vi "LHF.DB.Mongo.Bson.Waveform.vi"(0 "waveform":waveform(dbl), 5 "error in (no error)":errorcluster) -> (14 "BsonDocument":refnum<k24>, 19 "error out":errorcluster)   [LabVIEW 2013, in "LHF.DB.Mongo.lvclass"]
uses:
  LHF.DB.Mongo.lvclass
  C:/Users/Ricardo/Desktop/Projetos/LabVIEW-MongoDB/src/Driver/MongoDB.Bson.dll
  Driver/MongoDB.Bson.dll
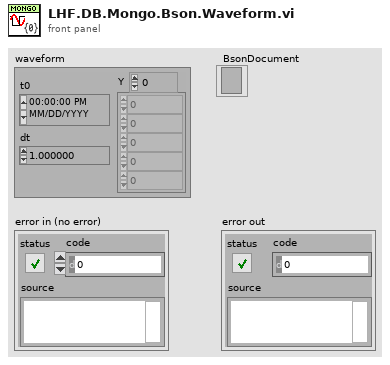
[diagram p1: front panel]
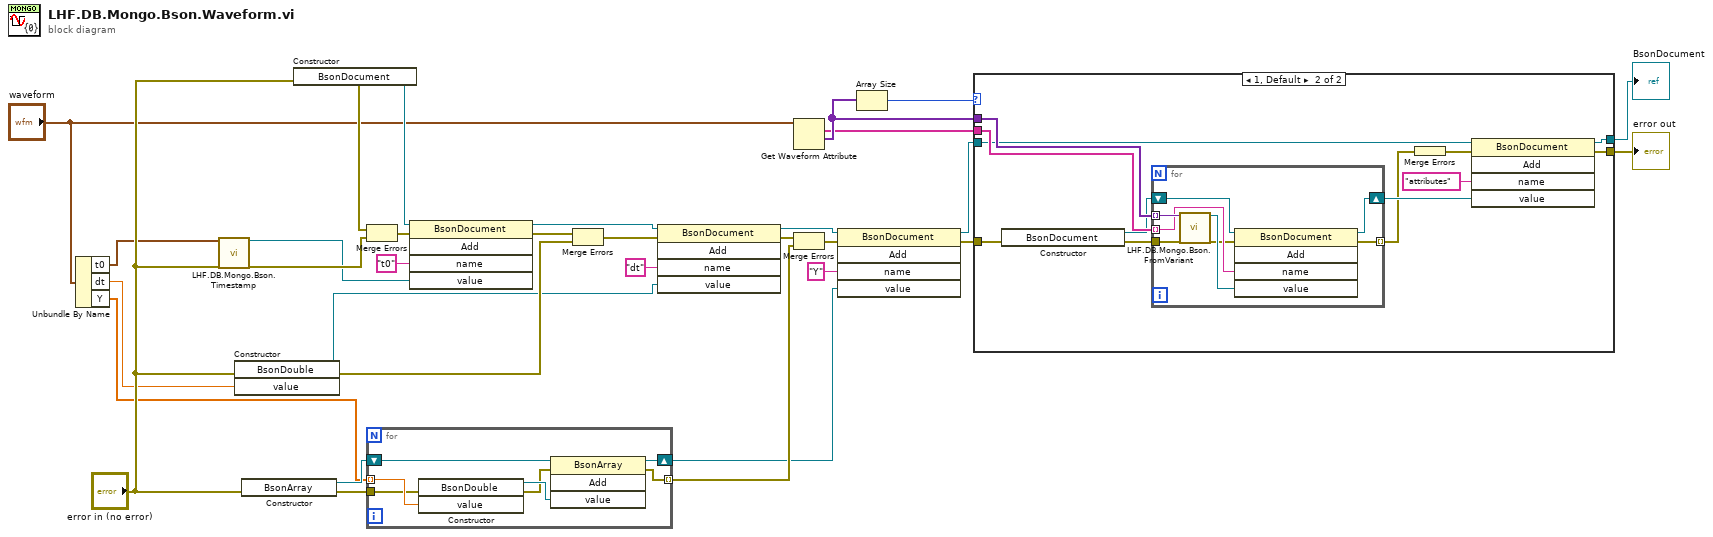
[diagram p0: block diagram]
diagram:
  n1 = Unbundle By Name("waveform") -> ("t0"=w5:timestamp, "dt"=w9:dbl, "Y"=w16:dbl[])
  n2 = call "LHF.DB.Mongo.Bson.Timestamp.vi"("t0"=w5, "error in (no error)"="error in (no error)") -> ("BsonString"=w8:refnum<k24>, "error out"=w25:errorcluster)  [unwired: 16 in]
  n3 = constructor class="BsonDouble"(error in="error in (no error)", "value"=w9) -> (reference out=w12:refnum<k24>, error out=w24:errorcluster)  [unwired: 2 in, 2 out]
  n4 = constructor class="BsonArray"(error in="error in (no error)") -> (reference out=w17:refnum<k24>, error out=w26:errorcluster)  [unwired: 2 in, 1 out]
  n5 = constructor class="BsonDocument"(error in="error in (no error)") -> (reference out=w6:refnum<k24>, error out=w31:errorcluster)  [unwired: 2 in, 1 out]
  n6 = Merge Errors(w31, w25) -> (w30:errorcluster)
  n7 = for {
    tunnel: w16 -> [w39] mode=indexing
    shift-right: [w36] -> w18
    shift-left: w17 -> [w38]
    tunnel: [w35] -> w22 mode=indexing
    tunnel: w26 -> [w34]
    n8 = constructor class="BsonDouble"(error in=w34, "value"=w39) -> (reference out=w37:refnum<k24>, error out=w33:errorcluster)  [unwired: 2 in, 2 out]
    n9 = invoke class="BsonArray" method="Add"(reference=w38, error in=w33, "value"=w37) -> (reference out=w36:refnum<k24>, error out=w35:errorcluster)  [unwired: 1 in, 2 out]
  }
  n10 = invoke class="BsonDocument" method="Add"(reference=w6, error in=w30, "name"="t0", "value"=w8) -> (reference out=w11:refnum<k24>, error out=w28:errorcluster)  [unwired: 1 in, 3 out]
  n11 = Merge Errors(w28, w24) -> (w27:errorcluster)
  n12 = invoke class="BsonDocument" method="Add"(reference=w11, error in=w27, "name"="dt", "value"=w12) -> (reference out=w15:refnum<k24>, error out=w29:errorcluster)  [unwired: 1 in, 3 out]
  n13 = Get Waveform Attribute(7:"waveform") -> (1:w3:variant[], 2:w2:string[])  [unwired: 3 in, 2 out]
  n14 = Merge Errors(w29, w22) -> (w23:errorcluster)
  n15 = invoke class="BsonDocument" method="Add"(reference=w15, error in=w23, "name"="Y", "value"=w18) -> (reference out=w14:refnum<k24>, error out=w21:errorcluster)  [unwired: 1 in, 3 out]
  n16 = Array Size(array=w3) -> (size(s)=w1:i32)
  n17 = case shown="1, Default" w1 {
    tunnel: w2 -> [_ w53]
    tunnel: w3 -> [_ w52]
    tunnel: w14 -> [w41 w48]
    tunnel: [w41 w47] -> w19
    tunnel: [w40 w43] -> w20
    tunnel: w21 -> [w40 w42]
    frame 0 {
    }
    frame 1, Default {
      n18 = constructor class="BsonDocument"(error in=w42) -> (reference out=w51:refnum<k24>, error out=w46:errorcluster)  [unwired: 2 in, 1 out]
      n19 = for {
        tunnel: w53 -> [w59] mode=indexing
        tunnel: w52 -> [w61] mode=indexing
        shift-right: [w57] -> w49
        shift-left: w51 -> [w58]
        tunnel: w46 -> [w56]
        tunnel: [w54] -> w45 mode=indexing
        n20 = call "LHF.DB.Mongo.Bson.FromVariant.vi"("Variant"=w61, "error IO"=w56) -> ("BsonValue"=w60:refnum<k24>, "error IO 2"=w55:errorcluster)  [unwired: 16 in]
        n21 = invoke class="BsonDocument" method="Add"(reference=w58, error in=w55, "name"=w59, "value"=w60) -> (reference out=w57:refnum<k24>, error out=w54:errorcluster)  [unwired: 1 in, 3 out]
      }
      n22 = Merge Errors(w45) -> (w44:errorcluster)
      n23 = invoke class="BsonDocument" method="Add"(reference=w48, error in=w44, "name"="attributes", "value"=w49) -> (reference out=w47:refnum<k24>, error out=w43:errorcluster)  [unwired: 1 in, 3 out]
    }
  }
  "error out" <- w20
  "BsonDocument" <- w19
